vi "Set Friction.vi"(7 "Viscous Friction":dbl, 8 "error in (no error)":errorcluster, 9 "Negative Coulomb Friction":dbl, 10 "Positive Coulomb Friction":dbl, 11 "Link in":refnum<class "NI_Robotics_Link.lvclass">) -> (0 "error out":errorcluster, 3 "Link out":refnum<class "NI_Robotics_Link.lvclass">)   [LabVIEW 2017, in "NI_Robotics_Link.lvclass"]
uses:
  <vilib>/robotics/Kinematics/Link/NI_Robotics_Link.lvclass
  <vilib>/robotics/Kinematics/Link/NI_Robotics_Link.lvclass/NI_Robotics_Link.ctl
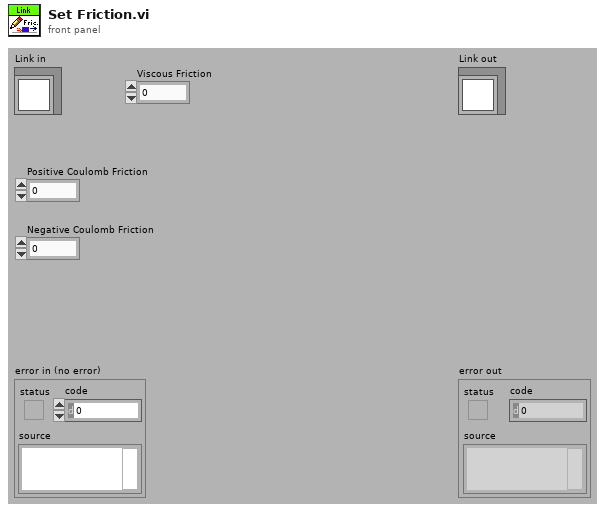
[diagram p1: front panel]
types:
  T1 = cluster{"Positive Coulomb Friction":dbl, "Negative Coulomb Friction":dbl}
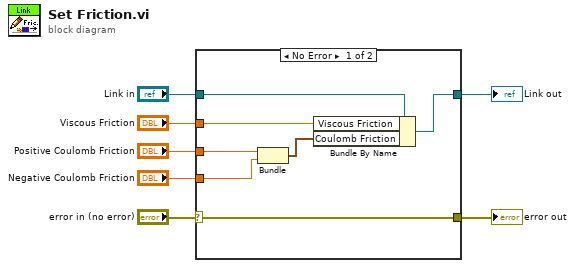
[diagram p0: block diagram]
diagram:
  n1 = case shown="No Error" "error in (no error)" {
    selector: "error in (no error)" -> [w14 w16]
    tunnel: [w14 w16] -> w6
    tunnel: [w8 w15] -> w4
    tunnel: "Link in" -> [w13 w15]
    tunnel: "Positive Coulomb Friction" -> [w11 _]
    tunnel: "Negative Coulomb Friction" -> [w10 _]
    tunnel: "Viscous Friction" -> [w9 _]
    frame No Error {
      n2 = Bundle("Positive Coulomb Friction"=w11, "Negative Coulomb Friction"=w10) -> (w12:T1)  [unwired: 1 in]
      n3 = Bundle By Name(cluster=w13, "Viscous Friction"=w9, "Coulomb Friction"=w12) -> (w8:refnum<class "NI_Robotics_Link.lvclass">)
    }
    frame Error {
    }
  }
  "error out" <- w6
  "Link out" <- w4
